vi "Stop Core.vi"(10 "final error code":i32, 11 "UI Actor in":refnum<class "UI Actor.lvclass">) -> (3 "UI Actor out":refnum<class "UI Actor.lvclass">)   [LabVIEW 2014, in "Device Test.lvlib" / "UI Actor.lvclass"]
doc: "(<B>Filename</B>: Actor Framework.lvlib:Actor.lvclass:Stop Core.vi)\n\nDefines what the actor does before it stops. Use the <B>final error code</B> input to determine whether the actor shut down in response to an error.\n\nBy default, this method does nothing. A descendant class may override it to define behavior, such as shutting down any processes the actor initiated in its override of the Actor Core method."
uses:
  UI Actor.lvclass
  UI Actor.lvclass/UI Actor.ctl
  <vilib>/ActorFramework/Actor/Actor.lvclass
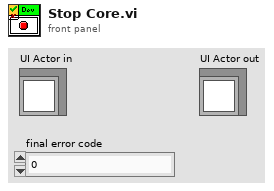
[diagram p1: front panel]
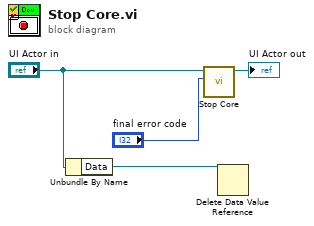
[diagram p0: block diagram]
diagram:
  n1 = Unbundle By Name("UI Actor in") -> ("Data"=w1:refnum<data-value>)
  n2 = call-parent "Stop Core.vi"("final error code"="final error code", "Actor in"="UI Actor in") -> ("Actor out"=→"UI Actor out":refnum<class "UI Actor.lvclass">)  [unwired: 9 in]
  n3 = Delete Data Value Reference(data value reference=w1) -> ()  [unwired: 1 in, 2 out]
